vi "Get BuildSpec Type.vi"(11 "Build Specification Name in":string) -> (1 "Build Spec Type":string, 2 "Found ?":bool, 3 "Build Specification Name out":string)   [LabVIEW 2020, in "LVLIBP CD XML Updater.lvlib"]
uses:
  LVLIBP CD XML Updater.lvlib
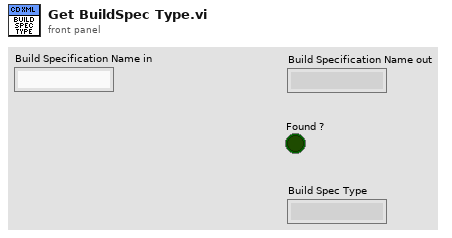
[diagram p1: front panel]
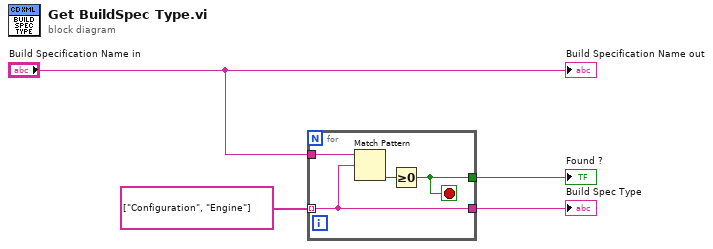
[diagram p0: block diagram]
diagram:
  n1 = for {
    tunnel: "Build Specification Name in" -> [w8]
    tunnel: string[] ["Configuration", "Engine"] -> [w6] mode=indexing
    tunnel: [w6] -> w1
    tunnel: [w5] -> w2
    stop <- w5 stop-if-true
    n2 = Match Pattern(string=w8, regular expression=w6) -> (offset past match=w7:i32)  [unwired: 1 in, 3 out]
    n3 = Greater Or Equal To 0?(x=w7) -> (x >= 0?=w5:bool)
  }
  "Found ?" <- w2
  "Build Spec Type" <- w1
  "Build Specification Name out" <- "Build Specification Name in"
